vi "LV message server.vi"() -> ()   [LabVIEW 2019]
uses:
  <vilib>/addons/zeromq/socket_type.ctl
  <vilib>/Waveform/WDTOps.llb/WDT Number of Waveform Samples DBL.vi
  <vilib>/addons/zeromq/zmq_context.lvclass
  <vilib>/addons/zeromq/zmq_socket.lvclass
  <vilib>/addons/zeromq/zeromq.lvlib
  <vilib>/measure/NI_MABase.lvlib
panel:
  out "Config":cluster{"Instrument":string, "Fs":dbl}
  out "size(s)":i32
  out "TX data":waveform(dbl)(graph)
  out "message history":string[](array[string])
  out "error out":errorcluster
  in  "Stop Button":bool
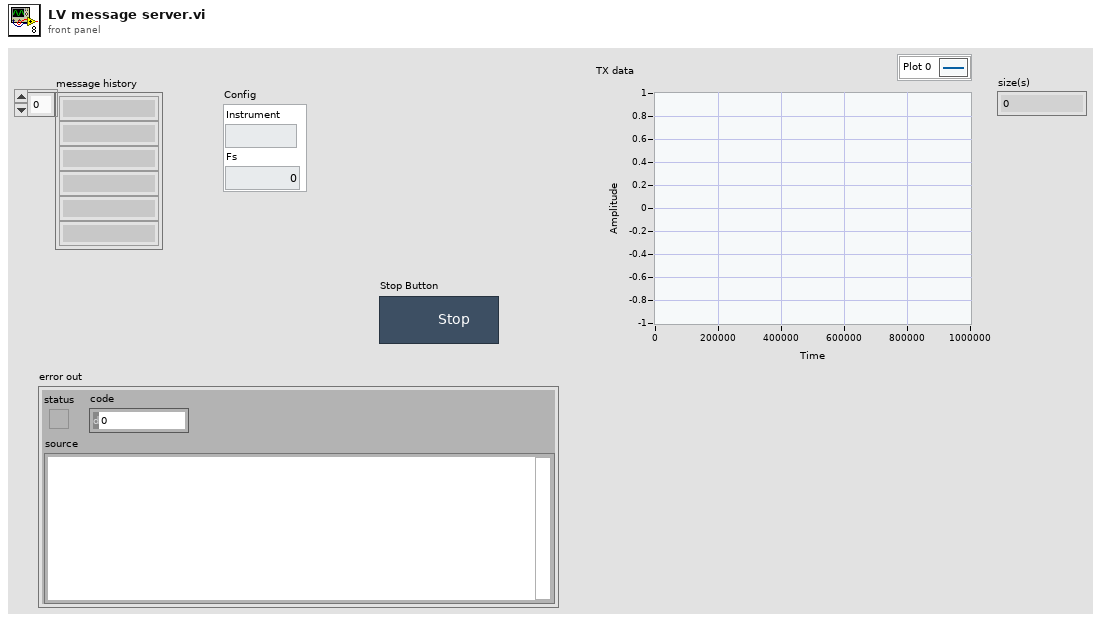
[diagram p1: front panel]
types:
  T1 = typedef "zeromq.lvlib/socket_type.ctl" = enum8{"ZMQ_PAIR", "ZMQ_PUB", "ZMQ_SUB", "ZMQ_REQ", "ZMQ_REP", "ZMQ_DEALER", "ZMQ_ROUTER", "ZMQ_PULL", "ZMQ_PUSH", "ZMQ_XPUB", "ZMQ_XSUB"}
  T2 = enum16{"big-endian, network order", "native, host order", "little-endian"}
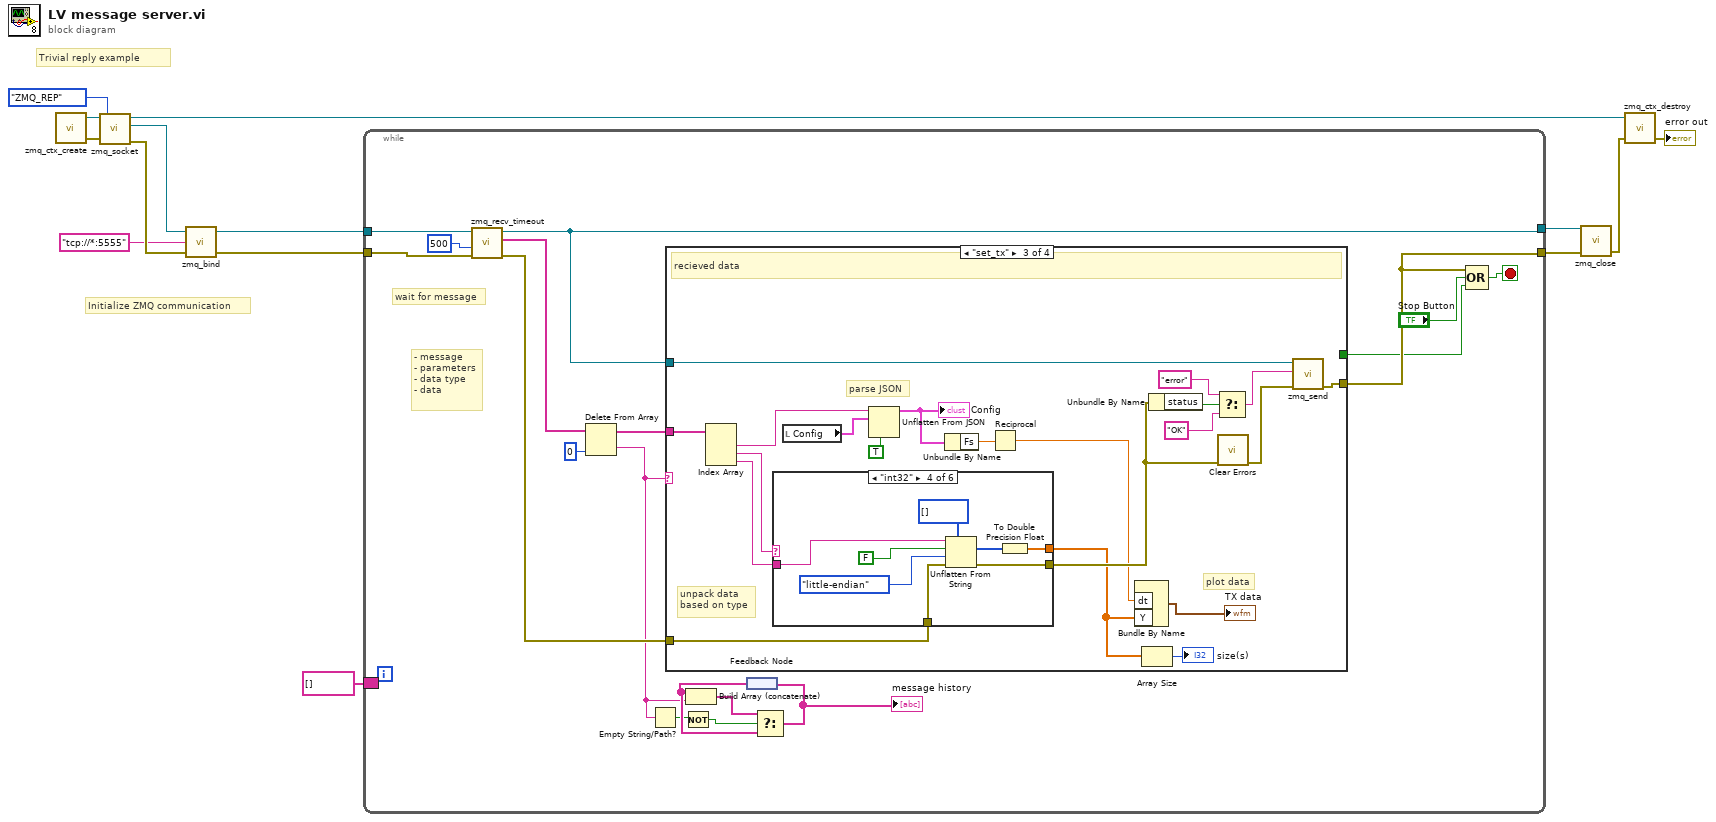
[diagram p0: block diagram]
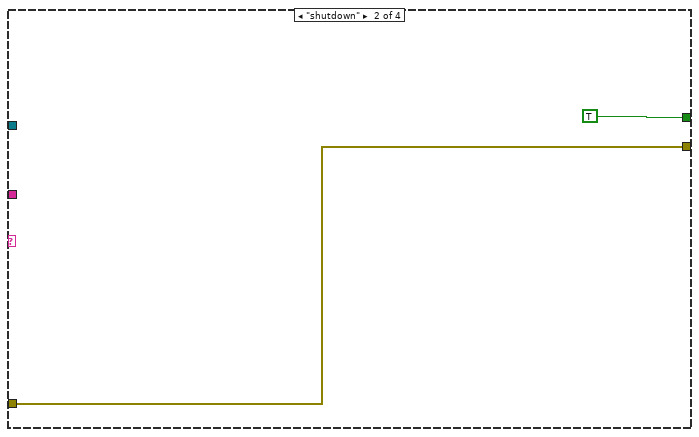
[diagram p3: hidden frame]
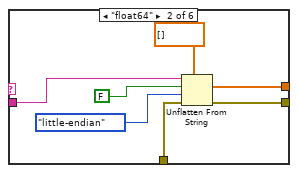
[diagram p5: hidden frame]
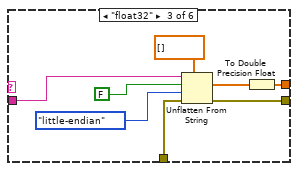
[diagram p6: hidden frame]
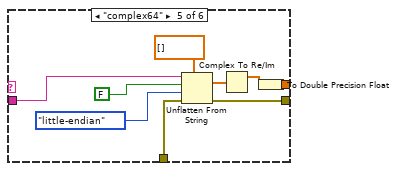
[diagram p7: hidden frame]
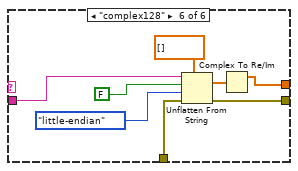
[diagram p8: hidden frame]
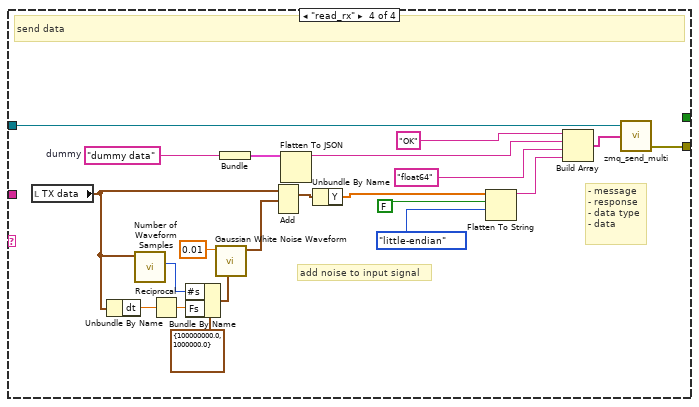
[diagram p9: hidden frame]
diagram:
  # "Initialize ZMQ communication"
  # "Trivial reply example"
  n1 = call <vilib>:"zmq_ctx_create.vi"() -> ("error out"=w12:errorcluster, "context out"=w11:refnum<class "zmq_context.lvclass">)  [unwired: 4 in]
  n2 = call <vilib>:"zmq_socket.vi"("error in"=w12, "socket type"=socket_type."ZMQ_REP", "context in"=w11) -> ("error out"=w14:errorcluster, "socket out"=w13:refnum<class "zmq_socket.lvclass">, "context out"=w5:refnum<class "zmq_context.lvclass">)  [unwired: 2 in]
  n3 = call <vilib>:"zmq_bind.vi"("error in"=w14, "endpoint"="tcp://*:5555", "socket in"=w13) -> ("error out"=w3:errorcluster, "socket out"=w4:refnum<class "zmq_socket.lvclass">)  [unwired: 1 in]
  n4 = while {
    tunnel: w4 -> [w32]
    tunnel: w3 -> [w31]
    tunnel: [w25] -> w8
    tunnel: [w29] -> w7
    border: string[] [] -> [_]
    stop <- w27 stop-if-true
    # "- message\n- parameters\n- data type\n- data"
    # "wait for message"
    n5 = call <vilib>:"zmq_recv_timeout.vi"("error in"=w31, "timeout (ms)"=u32 500, "socket in"=w32) -> ("error out"=w28:errorcluster, "parts"=w20:string[], "socket out"=w29:refnum<class "zmq_socket.lvclass">)  [unwired: 1 in, 1 out]
    n6 = Delete From Array(array=w20, index=0) -> (deleted portion=w17:string, array with subset deleted=w18:string[])  [unwired: 1 in]
    n7 = Empty String/Path?(string/path=w17) -> (empty?=w16:bool)
    n8 = case shown="\"set_tx\"" w17 {
      tunnel: w29 -> [_ _ w51 w116]
      tunnel: w18 -> [_ _ w56 _]
      tunnel: w28 -> [w33 w35 w55 _]
      tunnel: [w33 w35 w41 w107] -> w25
      tunnel: [_ TRUE _ _] -> w24
      frame Default {
      }
      frame "shutdown" {
      }
      frame "set_tx" {
        # "plot data"
        # "unpack data\nbased on type"
        # "parse JSON"
        # "recieved data"
        n9 = Index Array(array=w56) -> (element #1=w44:string, element #2=w52:string, element #3=w53:string)  [unwired: 3 in]
        n10 = case shown="\"int32\"" w52 {
          tunnel: w55 -> [w57 w63 w71 w79 w88 w96]
          tunnel: [w57 w61 w69 w77 w86 w94] -> w50
          tunnel: [_ w60 w65 w73 w81 w90] -> w38
          tunnel: w53 -> [_ w59 w67 w75 w85 w93]
          frame "False", Default {
          }
          frame "float64" {
            n11 = Unflatten From String(type=dbl[] [], binary string=w59, data includes array or string size? (T)=FALSE, byte order (0:big-endian, network order)=T2."little-endian", error in (no error)=w63) -> (value=w60:dbl[], error out=w61:errorcluster)  [unwired: 1 out]
          }
          frame "float32" {
            n12 = Unflatten From String(type=sgl[] [], binary string=w67, data includes array or string size? (T)=FALSE, byte order (0:big-endian, network order)=T2."little-endian", error in (no error)=w71) -> (value=w68:sgl[], error out=w69:errorcluster)  [unwired: 1 out]
            n13 = To Double Precision Float(number=w68) -> (double precision float=w65:dbl[])
          }
          frame "int32" {
            n14 = Unflatten From String(type=i32[] [], binary string=w75, data includes array or string size? (T)=FALSE, byte order (0:big-endian, network order)=T2."little-endian", error in (no error)=w79) -> (value=w76:i32[], error out=w77:errorcluster)  [unwired: 1 out]
            n15 = To Double Precision Float(number=w76) -> (double precision float=w73:dbl[])
          }
          frame "complex64" {
            n16 = Unflatten From String(type=csg[] [], binary string=w85, data includes array or string size? (T)=FALSE, byte order (0:big-endian, network order)=T2."little-endian", error in (no error)=w88) -> (value=w83:csg[], error out=w86:errorcluster)  [unwired: 1 out]
            n17 = Complex To Re/Im(x + iy=w83) -> (x=w82:sgl[])  [unwired: 1 out]
            n18 = To Double Precision Float(number=w82) -> (double precision float=w81:dbl[])
          }
          frame "complex128" {
            n19 = Unflatten From String(type=cdb[] [], binary string=w93, data includes array or string size? (T)=FALSE, byte order (0:big-endian, network order)=T2."little-endian", error in (no error)=w96) -> (value=w91:cdb[], error out=w94:errorcluster)  [unwired: 1 out]
            n20 = Complex To Re/Im(x + iy=w91) -> (x=w90:dbl[])  [unwired: 1 out]
          }
        }
        n21 = local read "Config"() -> (w43:cluster{"Instrument":string, "Fs":dbl})
        n22 = Unflatten From JSON(JSON string=w44, type and defaults=w43, default null elements? (F)=TRUE) -> (value=w40:cluster{"Instrument":string, "Fs":dbl})  [unwired: 4 in, 1 out]
        "Config" <- w40
        n23 = Unbundle By Name(w40) -> ("Fs"=w39:dbl)
        n24 = Reciprocal(x=w39) -> (1/x=w37:dbl)
        n25 = Bundle By Name("dt"=w37, "Y"=w38) -> (→"TX data":waveform(dbl))  [unwired: 1 in]
        n26 = Array Size(array=w38) -> (size(s)=→"size(s)":i32)
        n27 = Unbundle By Name(w50) -> ("status"=w49:bool)
        n28 = Select(t="error" ("data"), s=w49, f="OK" ("data")) -> (s? t:f=w46:string)
        n29 = call <vilib>:"Clear Errors.vi"("error in (no error)"=w50) -> ("error out"=w47:errorcluster)  [unwired: 5 in, 1 out]
        n30 = call <vilib>:"zmq_send.vi"("error in"=w47, "data"=w46, "socket in"=w51) -> ("error out"=w41:errorcluster)  [unwired: 4 in, 1 out]
      }
      frame "read_rx" {
        w112 = "dummy data"  # dummy
        # "add noise to input signal"
        # "- message\n- response\n- data type\n- data"
        # "send data"
        n31 = local read "TX data"() -> (w100:waveform(dbl))
        n32 = Unbundle By Name(w100) -> ("dt"=w98:dbl)
        n33 = call-poly <vilib>:"Number of Waveform Samples.vi"("waveform in"=w100) -> ("number of samples"=w104:i32)  [unwired: 8 in, 2 out]
        n34 = Reciprocal(x=w98) -> (1/x=w99:dbl)
        n35 = Bundle By Name(cluster=cluster{"Fs":dbl, "#s":dbl} {"Fs"=100000000.0, "#s"=1000000.0} ("sampling info"), "#s"=w104, "Fs"=w99) -> (w105:cluster{"Fs":dbl, "#s":dbl})
        n36 = call <vilib>:"Gaussian White Noise Waveform.vi"("sampling info"=w105, "standard deviation"=0.01) -> ("signal out"=w103:waveform(dbl))  [unwired: 8 in, 1 out]
        n37 = Bundle("dummy"=w112) -> (w108:cluster{"dummy":string})  [unwired: 1 in]
        n38 = Add(1:w103, 2:w100) -> (0:w102:waveform(dbl))  [unwired: 1 in, 1 out]
        n39 = Flatten To JSON(anything=w108) -> (JSON string=w109:string)  [unwired: 2 in, 1 out]
        n40 = Unbundle By Name(w102) -> ("Y"=w101:dbl[])
        n41 = Flatten To String(anything=w101, prepend array or string size? (T)=FALSE, byte order (0:big-endian, network order)=T2."little-endian") -> (data string=w110:string)  [unwired: 1 in, 2 out]
        n42 = Build Array("OK" ("element"), w109, "float64" ("element"), w110) -> (w118:string[])
        n43 = call <vilib>:"zmq_send_multi.vi"("parts"=w118, "socket in"=w116) -> ("error out"=w107:errorcluster)  [unwired: 2 in, 1 out]
      }
    }
    n44 = Not(x=w16) -> (.not. x?=w15:bool)
    n45 = feedback #1() -> (w21:string[])
    n46 = Build Array (concatenate)(w21, w17) -> (w23:string[])
    n47 = Select(t=w23, s=w15, f=w21) -> (s? t:f=w22:string[])
    "message history" <- w22
    n48 = feedback-in #1(w22) -> ()
    n49 = Compound Arithmetic op=OR(w25, "Stop Button", w24) -> (w27:bool)
  }
  n50 = call <vilib>:"zmq_close.vi"("error in"=w8, "socket"=w7) -> ("error out"=w6:errorcluster)  [unwired: 3 in]
  n51 = call <vilib>:"zmq_ctx_destroy.vi"("error in"=w6, "context in"=w5) -> ("error out"=→"error out":errorcluster)  [unwired: 3 in]
